vi "UV_TemplateNo.vi"(6 "A/M (F:autoP)":bool, 7 "R/W (F:read)":bool, 8 "error in (no error)":errorcluster, 10 "template_set":T1, 11 "VISA resource":refnum<visa-resource-name>="COM5") -> (0 "error out":errorcluster, 2 "response":u8[](array[numeric]), 3 "VISA resource out":refnum<visa-resource-name>, 5 "Err?":bool)   [LabVIEW 2018]
uses:
  TypeDef/UVLed_func.ctl
  TypeDef/UVLed_channel.ctl
  low_level/convert/Gen_UV_CMD (SubVI).vi
  low_level/convert/CMD_SUM (SubVI).vi
  low_level/VISA query.vi
panel:
  # "For ManualPro and AutoPro Only"
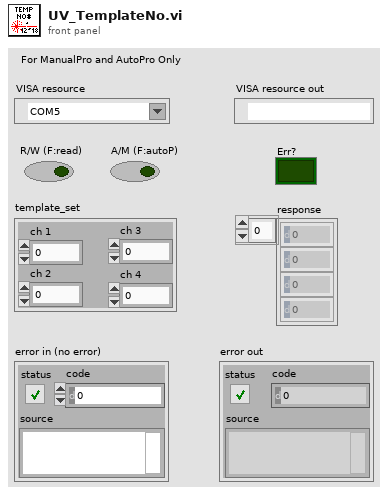
[diagram p1: front panel]
types:
  T1 = cluster{"ch 1":u8, "ch 2":u8, "ch 3":u8, "ch 4":u8}
  T2 = typedef "UVLed_func.ctl" = u16
  T3 = typedef "UVLed_channel.ctl" = u16
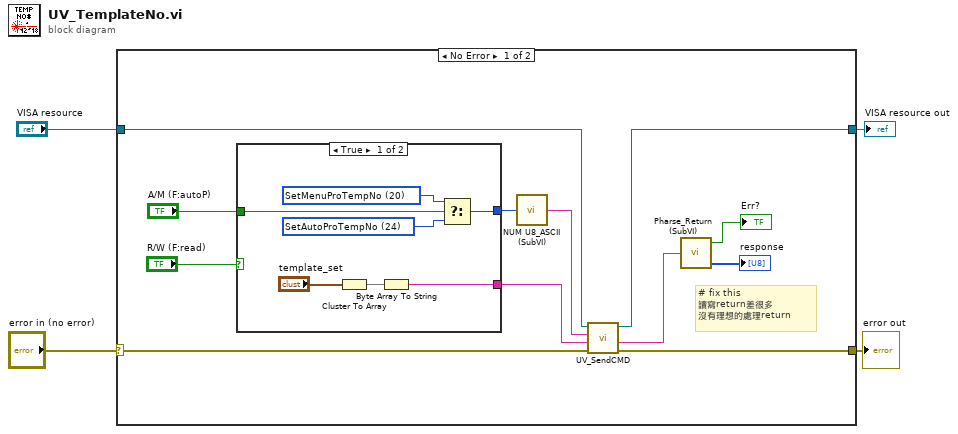
[diagram p0: block diagram]
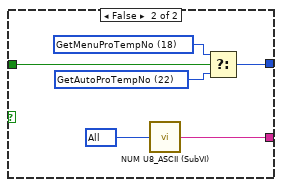
[diagram p2: hidden frame]
diagram:
  n1 = case shown="No Error" "error in (no error)" {
    selector: "error in (no error)" -> [w13 w31]
    tunnel: [w12 w31] -> w3
    tunnel: "VISA resource" -> [w14 w30]
    tunnel: [w10 w30] -> w1
    frame No Error {
      # "# fix this\n讀寫return差很多\n沒有理想的處理return"
      n2 = case shown="True" "R/W (F:read)" {
        tunnel: [w23 w29] -> w16
        tunnel: "A/M (F:autoP)" -> [w22 w26]
        tunnel: [w17 w25] -> w7
        frame True {
          w20 = T2 24 items=["GetAllStatus"=0, "LightOn"=2, "LightOff"=4, "AllForceOff"=6, "GetMenuChnPara"=10, "SetMenuChnPara"=12, "GetAutoChnPara"=14, "SetAutoChnPara"=16, "GetMenuProTempNo"=18, "SetMenuProTempNo"=20, "GetAutoProTempNo"=22, "SetAutoProTempNo"=24, "GetTemplatePara"=26, "SetTemplatePara"=28, "GetMode"=30, "SetMode"=32] ("Function")
          w21 = T2 20 items=["GetAllStatus"=0, "LightOn"=2, "LightOff"=4, "AllForceOff"=6, "GetMenuChnPara"=10, "SetMenuChnPara"=12, "GetAutoChnPara"=14, "SetAutoChnPara"=16, "GetMenuProTempNo"=18, "SetMenuProTempNo"=20, "GetAutoProTempNo"=22, "SetAutoProTempNo"=24, "GetTemplatePara"=26, "SetTemplatePara"=28, "GetMode"=30, "SetMode"=32] ("Function")
          n3 = Cluster To Array(cluster="template_set") -> (array=w18:u8[])
          n4 = Byte Array To String(unsigned byte array=w18) -> (string=w17:string)
          n5 = Select(t=w21, s=w22, f=w20) -> (s? t:f=w23:T2)
        }
        frame False {
          w27 = T2 22 items=["GetAllStatus"=0, "LightOn"=2, "LightOff"=4, "AllForceOff"=6, "GetMenuChnPara"=10, "SetMenuChnPara"=12, "GetAutoChnPara"=14, "SetAutoChnPara"=16, "GetMenuProTempNo"=18, "SetMenuProTempNo"=20, "GetAutoProTempNo"=22, "SetAutoProTempNo"=24, "GetTemplatePara"=26, "SetTemplatePara"=28, "GetMode"=30, "SetMode"=32] ("Function")
          w24 = T3 255 items=["All"=255, "CH1"=1, "CH2"=2, "CH3"=3, "CH4"=4] ("CHN")
          w28 = T2 18 items=["GetAllStatus"=0, "LightOn"=2, "LightOff"=4, "AllForceOff"=6, "GetMenuChnPara"=10, "SetMenuChnPara"=12, "GetAutoChnPara"=14, "SetAutoChnPara"=16, "GetMenuProTempNo"=18, "SetMenuProTempNo"=20, "GetAutoProTempNo"=22, "SetAutoProTempNo"=24, "GetTemplatePara"=26, "SetTemplatePara"=28, "GetMode"=30, "SetMode"=32] ("Function")
          n6 = call "NUM U8_ASCII (SubVI).vi"("Numeric"=w24) -> ("String out"=w25:string)
          n7 = Select(t=w28, s=w26, f=w27) -> (s? t:f=w29:T2)
        }
      }
      n8 = call "NUM U8_ASCII (SubVI).vi"("Numeric"=w16) -> ("String out"=w15:string)
      n9 = call "UV_SendCMD.vi"("error in"=w13, "value"=w7, "function"=w15, "VISA resource name"=w14) -> ("error out"=w12:errorcluster, "response"=w11:string, "VISA resource name out"=w10:refnum<visa-resource-name>)  [unwired: 5 in]
      n10 = call "Pharse_Return (SubVI).vi"("buffer in"=w11) -> ("byte array"=→"response":u8[], "Err?"=→"Err?":bool)  [unwired: 2 in, 1 out]
    }
    frame Error {
    }
  }
  "error out" <- w3
  "VISA resource out" <- w1
